vi "convert--tour to string (minimal format).vi"(1 "tour":T1[](array[typedef])) -> (0 "tour (minimal format)":string)   [LabVIEW 2020, in "main.lvlib"]
doc: "Converts the knight tour (array of chessboard_index) to a \"minimal\" format string (e.g. a1-c2-e3-g4-h6-g8-e7-c8-a7-b5-d6-f7-.....-a5-b3-c5)."
uses:
  main.lvlib
  core/core_data/chessboard_index.ctl
  core/core.lvlib
  core/core_data/core_data.lvlib
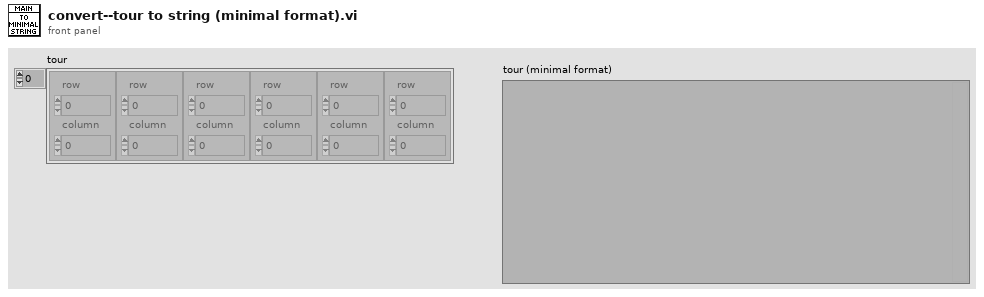
[diagram p1: front panel]
types:
  T1 = typedef "core.lvlib/core_data.lvlib/chessboard_index.ctl" = cluster{"row":u8, "column":u8}
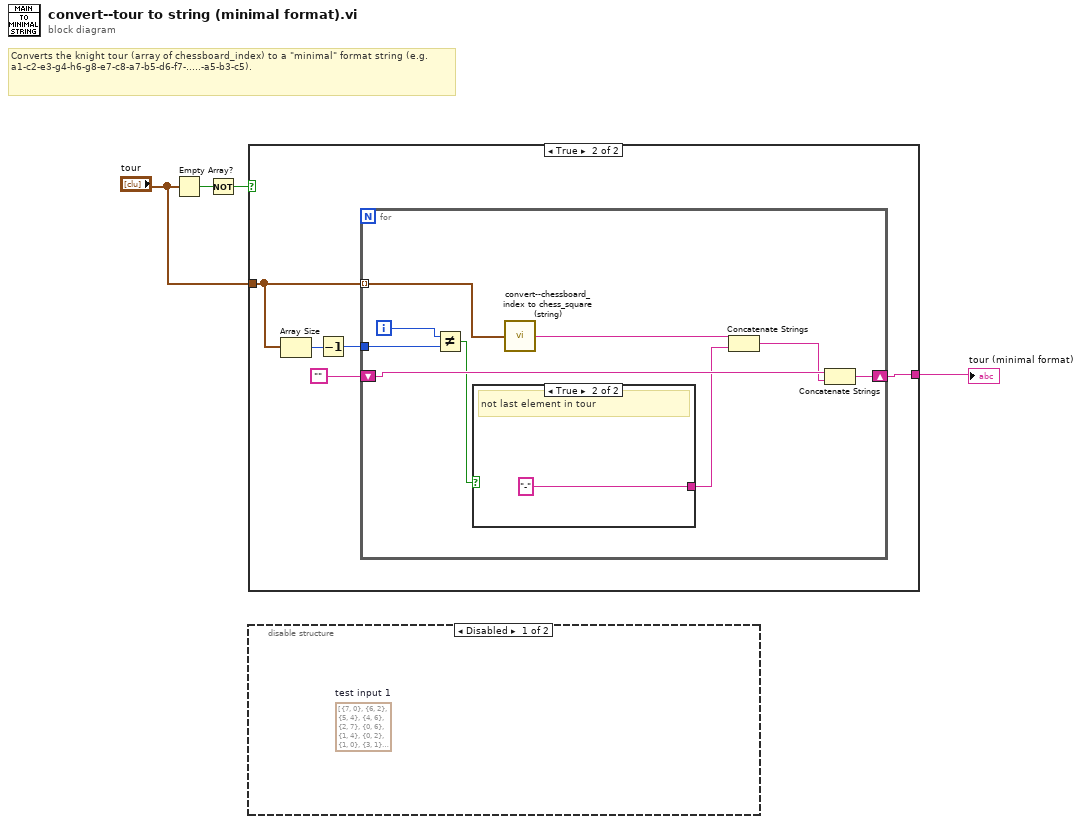
[diagram p0: block diagram]
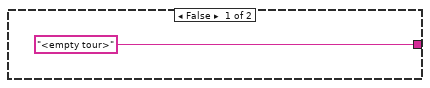
[diagram p3: hidden frame]
diagram:
  # "Converts the knight tour (array of chessboard_index) to a \"minimal\" format string (e.g. a1-c2-e3-g4-h6-g8-e7-c8-a7-b5-d6-f7-.....-a5-b3-c5)."
  n1 = Empty Array?(array="tour") -> (empty?=w4:bool)
  n2 = Not(x=w4) -> (.not. x?=w3:bool)
  n3 = case shown="True" w3 {
    tunnel: ["<empty tour>" w6] -> w2
    tunnel: "tour" -> [_ w9]
    frame False {
    }
    frame True {
      n4 = Array Size(array=w9) -> (size(s)=w8:i32)
      n5 = Decrement(x=w8) -> (x-1=w7:i32)
      n6 = for {
        tunnel: w9 -> [w17] mode=indexing
        tunnel: w7 -> [w18]
        shift-right: [w15] -> w6
        shift-left: "" -> [w16]
        i -> [w19]
        n7 = Not Equal?(x=w19, y=w18) -> (x != y?=w13:bool)
        n8 = case shown="True" w13 {
          tunnel: [_ "-"] -> w12
          frame False {
          }
          frame True {
            # "not last element in tour"
          }
        }
        n9 = call "convert--chessboard_index to chess_square (string).vi"("chessboard_index"=w17) -> ("chess square (string)"=w14:string)
        n10 = Concatenate Strings(w14, w12) -> (w11:string)
        n11 = Concatenate Strings(w16, w11) -> (w15:string)
      }
    }
  }
  "tour (minimal format)" <- w2
  n12 = disable-structure shown="Disabled" {
    frame Disabled {
      (unwired) T1[] [{"row"=7, "column"=0}, {"row"=6, "column"=2}, {"row"=5, "column"=4}, {"row"=4, "column"=6}, {"row"=2, "column"=7}, {"row"=0, "column"=6}, {"row"=1, "column"=4}, {"row"=0, "column"=2}, {"row"=1, "column"=0}, {"row"=3, "column"=1}, {"row"=2, "column"=3}, {"row"=1, "column"=5}, {"row"=0, "column"=7}, {"row"=2, "column"=6}, {"row"=0, "column"=5}, {"row"=1, "column"=3}, {"row"=0, "column"=1}, {"row"=2, "column"=0}, {"row"=1, "column"=2}, {"row"=0, "column"=4}, {"row"=2, "column"=5}, {"row"=1, "column"=7}, {"row"=3, "column"=6}, {"row"=2, "column"=4}, {"row"=1, "column"=6}, {"row"=3, "column"=5}, {"row"=4, "column"=3}, {"row"=2, "column"=2}, {"row"=0, "column"=3}, {"row"=1, "column"=1}, {"row"=3, "column"=0}, {"row"=5, "column"=1}, {"row"=3, "column"=2}]  # test input 1
    }
    frame Enabled {
    }
  }
